vi "Write # holes in one.vi"(8 "error in (no error)":errorcluster, 10 "# holes in one":i32, 11 "Golf Player in":refnum<class "Golf Player.lvclass">) -> (0 "error out":errorcluster, 3 "Golf Player out":refnum<class "Golf Player.lvclass">)   [LabVIEW 2019, in "Golf Player.lvclass"]
uses:
  Golf Player.lvclass
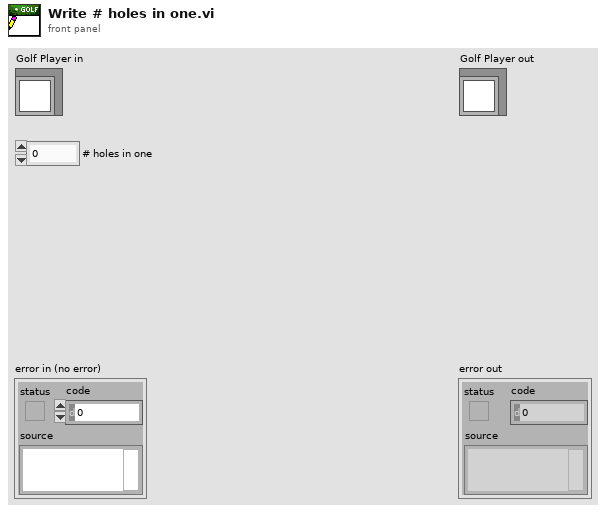
[diagram p1: front panel]
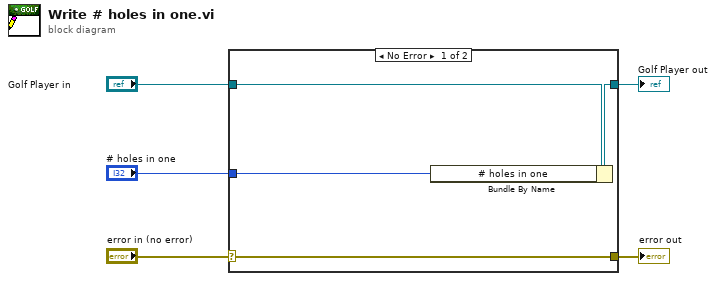
[diagram p0: block diagram]
diagram:
  n1 = case shown="No Error" "error in (no error)" {
    selector: "error in (no error)" -> [w9 w10]
    tunnel: [w9 w10] -> w4
    tunnel: [w7 w11] -> w2
    tunnel: "Golf Player in" -> [w8 w11]
    tunnel: "# holes in one" -> [w6 _]
    frame No Error {
      n2 = Bundle By Name(cluster=w8, "# holes in one"=w6) -> (w7:refnum<class "Golf Player.lvclass">)
    }
    frame Error {
    }
  }
  "error out" <- w4
  "Golf Player out" <- w2
